vi "Close.vi"(8 "error in (no error)":errorcluster, 11 "BiStableShutter in":refnum<class "BiStableShutter.lvclass">) -> (0 "error out":errorcluster, 3 "BiStableShutter out":refnum<class "BiStableShutter.lvclass">)   [LabVIEW 2016, in "BiStableShutter.lvclass"]
uses:
  BiStableShutter.lvclass
  Shutter.lvclass
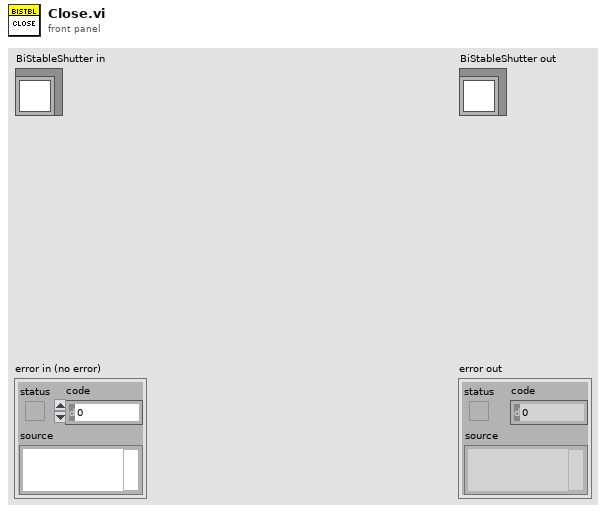
[diagram p1: front panel]
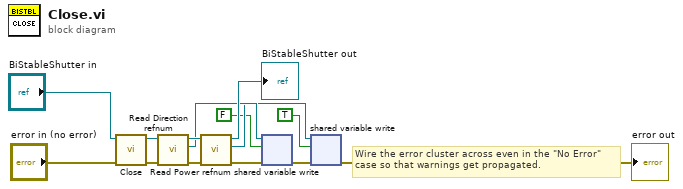
[diagram p0: block diagram]
diagram:
  # "Wire the error cluster across even in the \"No Error\"\ncase so that warnings get propagated."
  n1 = call-parent "Close.vi"("error in (no error)"="error in (no error)", "Shutter in"="BiStableShutter in") -> ("error out"=w3:errorcluster, "Shutter out"=w4:refnum<class "BiStableShutter.lvclass">)  [unwired: 8 in]
  n2 = call-dynamic "Read Direction refnum.vi"("error in (no error)"=w3, "BiStableShutter in"=w4) -> ("error out"=w11:errorcluster, "Direction refnum"=w10:refnum<k21>, "BiStableShutter out"=w12:refnum<class "BiStableShutter.lvclass">)  [unwired: 7 in]
  n3 = call-dynamic "Read Power refnum.vi"("error in (no error)"=w11, "BiStableShutter in"=w12) -> ("error out"=w8:errorcluster, "Power refnum"=w9:refnum<k21>, "BiStableShutter out"=→"BiStableShutter out":refnum<class "BiStableShutter.lvclass">)  [unwired: 7 in]
  n4 = shared-variable-write(w10, w8, FALSE ("data in")) -> (w7:errorcluster)  [unwired: 1 out]
  n5 = shared-variable-write(w9, w7, TRUE) -> (→"error out":errorcluster)  [unwired: 1 out]
